vi "ws_edittest import sequence.vi"(6 "User":T3, 8 "error in (no error)":errorcluster, 9 "UploadedFilesList":T1(array[cluster]), 10 "Filename":string, 11 "Connection Refnum":T2) -> (0 "error out":errorcluster, 2 "Sequence Record":T4, 3 "Connection Refnum":T2)   [LabVIEW 2011]
uses:
  server/database/Sequences/Sequence Record.ctl
  server/database/Users/User Record.ctl
  SI.LIB/ODBC/SQL Controls/Connection Refnum.ctl
  <vilib>/Utility/config.llb/NI_LVConfig.lvlib
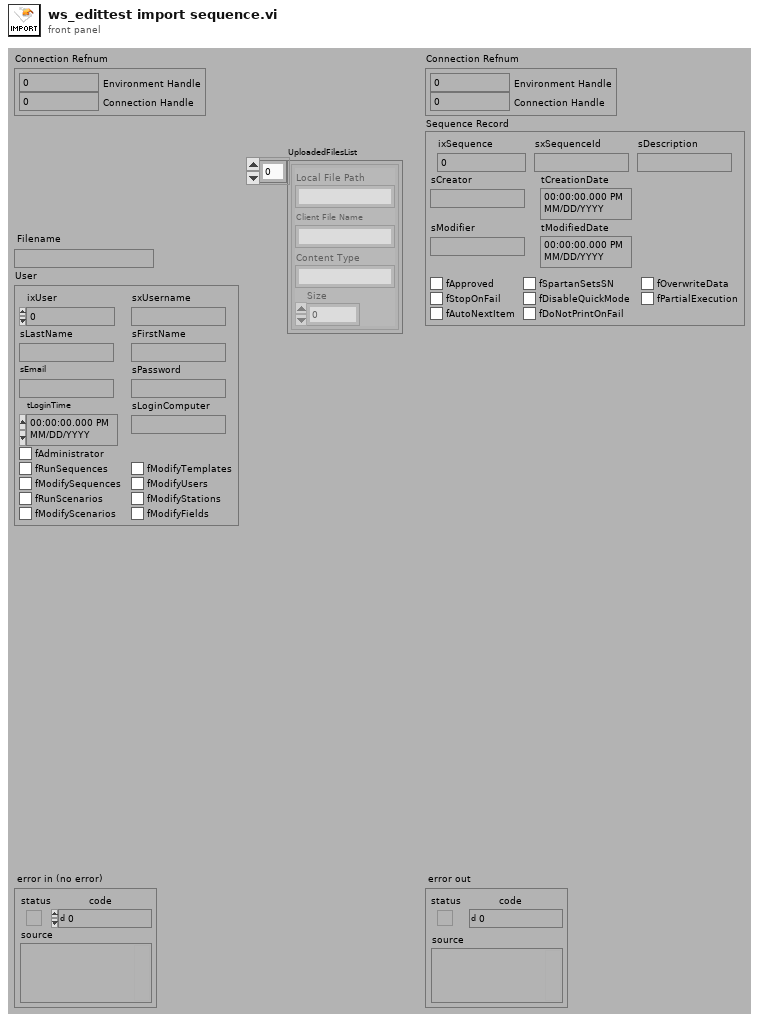
[diagram p1: front panel]
types:
  T1 = cluster{"Local File Path":string, "Client File Name":string, "Content Type":string, "Size":u32}[]
  T2 = typedef "Connection Refnum.ctl" = cluster{"Environment Handle":i32, "Connection Handle":i32}
  T3 = typedef "User Record.ctl" = cluster{"ixUser":i32, "sxUsername":string, "sLastName":string, "sFirstName":string, "sEmail":string, "sPassword":string, "tLoginTime":timestamp, "sLoginComputer":string, "fAdministrator":bool, "fRunSequences":bool, "fModifySequences":bool, "fRunScenarios":bool, "fModifyScenarios":bool, "fModifyTemplates":bool, "fModifyUsers":bool, "fModifyStations":bool, "fModifyFields":bool}
  T4 = typedef "Sequence Record.ctl" = cluster{"ixSequence":i32, "sxSequenceId":string, "sDescription":string, "sCreator":string, "tCreationDate":timestamp, "sModifier":string, "tModifiedDate":timestamp, "fApproved":bool, "fSpartanSetsSN":bool, "fOverwriteData":bool, "fStopOnFail":bool, "fDisableQuickMode":bool, "fPartialExecution":bool, "fAutoNextItem":bool, "fDoNotPrintOnFail":bool}
  T5 = typedef "NI_LVConfig.lvlib/Config Data RefNum.ctl" = refnum<k1>
  T6 = typedef "Step Record.ctl" = cluster{"ixStep":i32, "sxSequenceId":string, "sxTestId":string, "iIndex":i32, "iRepeat":i32, "iQuickMode":i32, "sTag":string, "sDatasheetsCSV":string, "bConfiguration":string}
  T7 = typedef "Field Record.ctl" = cluster{"ixField":i32, "iSequenceOrder":i32, "sxFieldId":string, "sxSequenceId":string, "sDisplayName":string, "sValue":string, "sUnits":string, "nDataType":T8, "nNextItem":T9, "fSystem":bool, "fSystemValue":bool, "fRequired":bool, "fSetAtTest":bool, "fTestField":bool, "fDeleted":bool, "fIndexed":bool, "fFreeList":bool}
  T8 = typedef "Field DataTypes.ctl" = enum32{"text", "numeric", "list", "timestamp", "boolean"}
  T9 = typedef "Field NextItem.ctl" = enum32{"Reset", "Retain", "Auto-Increment"}
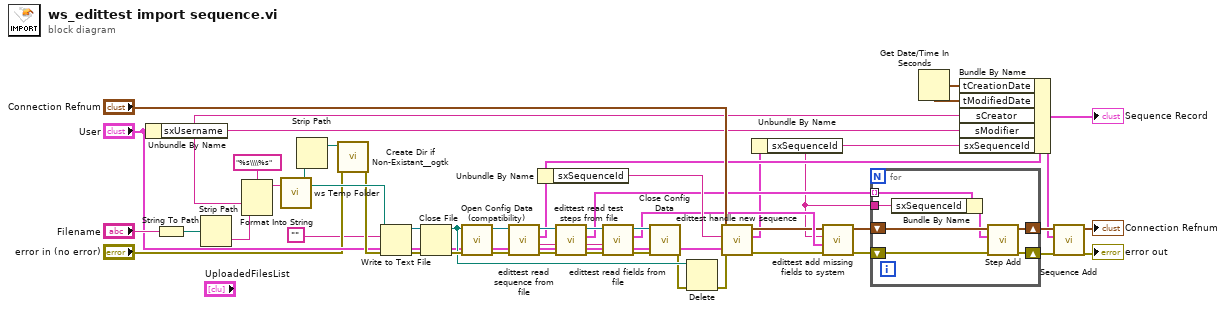
[diagram p0: block diagram]
diagram:
  n1 = Unbundle By Name("User") -> ("sxUsername"=w16:string)
  n2 = String To Path(string="Filename") -> (path=w24:path)
  n3 = Strip Path(path=w24) -> (name=w22:string)  [unwired: 1 out]
  n4 = Format Into String(format string="%s\\\\%s" ("Relative Path (\"\" - Folder)"), w16, w22) -> (resulting string=w32:string)  [unwired: 2 in, 1 out]
  n5 = call "ws Temp Folder.vi"("Relative Path (\"\")"=w32) -> ("Temp Folder"=w29:path)  [unwired: 2 in]
  n6 = Strip Path(path=w29) -> (stripped path=w30:path)  [unwired: 1 out]
  n7 = call <userlib>:"Create Dir if Non-Existant__ogtk.vi"("error in (no error)"="error in (no error)", "Directory Path"=w30) -> ("error out"=w28:errorcluster)  [unwired: 1 in, 8 out]
  n8 = Write to Text File(file (use dialog)=w29, text="", error in=w28) -> (refnum out=w34:refnum<file>, error out=w36:errorcluster)  [unwired: 2 out]
  n9 = Close File(refnum=w34, error in=w36) -> (path=w21:path, error out=w35:errorcluster)
  n10 = call <vilib>:"Open Config Data (compatibility).vi"("error in (no error)"=w35, "configuration file path"=w21) -> ("error out"=w44:errorcluster, "refnum"=w31:T5)  [unwired: 7 in, 1 out]
  n11 = call "edittest read sequence from file.vi"("error in (no error)"=w44, "File Refnum In"=w31) -> ("error out"=w43:errorcluster, "Version"=w37:string, "Sequence Record"=w25:T4, "File Refnum Out"=w42:T5)  [unwired: 6 out]
  n12 = Unbundle By Name(w25) -> ("sxSequenceId"=w26:string)
  n13 = call "edittest read test steps from file.vi"("error in (no error)"=w43, "Version"=w37, "File Refnum In"=w42) -> ("error out"=w41:errorcluster, "Sequence Steps"=w13:T6[], "File Refnum Out"=w40:T5)  [unwired: 6 out]
  n14 = call "edittest read fields from file.vi"("error in (no error)"=w41, "Version"=w37, "File Refnum In"=w40) -> ("error out"=w38:errorcluster, "Sequence Fields"=w17:T7[], "File Refnum Out"=w39:T5)  [unwired: 6 out]
  n15 = call <vilib>:"Close Config Data.vi"("error in (no error)"=w38, "refnum"=w39) -> ("error out"=w20:errorcluster)  [unwired: 1 in, 8 out]
  n16 = Delete(path (use dialog)=w21, error in=w20) -> (error out=w19:errorcluster)  [unwired: 5 out]
  n17 = call "edittest handle new sequence.vi"("User Information"="User", "error in (no error)"=w19, "New Name Suggestion\n(empty - \"Username Sequence N\")"=w26, "Connection Refnum"="Connection Refnum") -> ("error out"=w18:errorcluster, "New Sequence Record"=w9:T4, "Connection Refnum"=w10:T2)  [unwired: 5 out]
  n18 = Unbundle By Name(w9) -> ("sxSequenceId"=w3:string)
  n19 = call "edittest add missing fields to system.vi"("error in (no error)"=w18, "Fields"=w17, "sxSequenceId (\"\")"=w3, "Connection Refnum"=w10) -> ("error out"=w11:errorcluster, "Connection Refnum"=w12:T2)  [unwired: 6 out]
  n20 = for {
    tunnel: w13 -> [w47] mode=indexing
    shift-right: [w48] -> w8
    shift-left: w11 -> [w50]
    shift-right: [w49] -> w6
    shift-left: w12 -> [w51]
    tunnel: w3 -> [w46]
    n21 = Bundle By Name(cluster=w47, "sxSequenceId"=w46) -> (w45:T6)
    n22 = call "Step Add.vi"("error in (no error)"=w50, "Step Record"=w45, "Connection Refnum"=w51) -> ("error out"=w48:errorcluster, "Connection Refnum"=w49:T2)  [unwired: 7 out]
  }
  n23 = Get Date/Time In Seconds() -> (seconds since 1Jan1904=w15:timestamp)
  n24 = Bundle By Name(cluster=w25, "tCreationDate"=w15, "tModifiedDate"=w15, "sCreator"=w16, "sModifier"=w16, "sxSequenceId"=w3) -> (w4:T4)
  "Sequence Record" <- w4
  n25 = call "Sequence Add.vi"("error in (no error)"=w8, "Sequence Record"=w4, "Connection Refnum"=w6) -> ("error out"=→"error out":errorcluster, "Connection Refnum"=→"Connection Refnum":T2)  [unwired: 7 out]
